vi "test git.vi"() -> ()   [LabVIEW 2023]
panel:
  out "Numeric 2":dbl
  in  "Numeric":dbl
  # "DEV1 and DEV2"
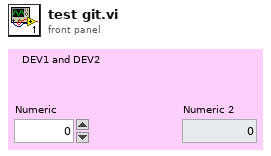
[diagram p1: front panel]
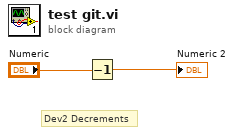
[diagram p0: block diagram]
diagram:
  # "Dev2 Decrements"
  n1 = Decrement(x="Numeric") -> (x-1=→"Numeric 2":dbl)
